vi "Win_Handler.vi"() -> ()   [LabVIEW 2025]
panel:
  out "Error Out":errorcluster
  in  "Error In":errorcluster
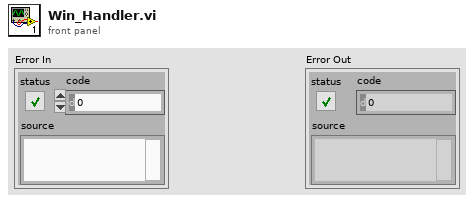
[diagram p1: front panel]
types:
  T1 = typedef "Queue_Data.ctl" = cluster{"CMD":string, "Data":variant}
  T2 = typedef "IMAQ Image.ctl" = refnum<image>
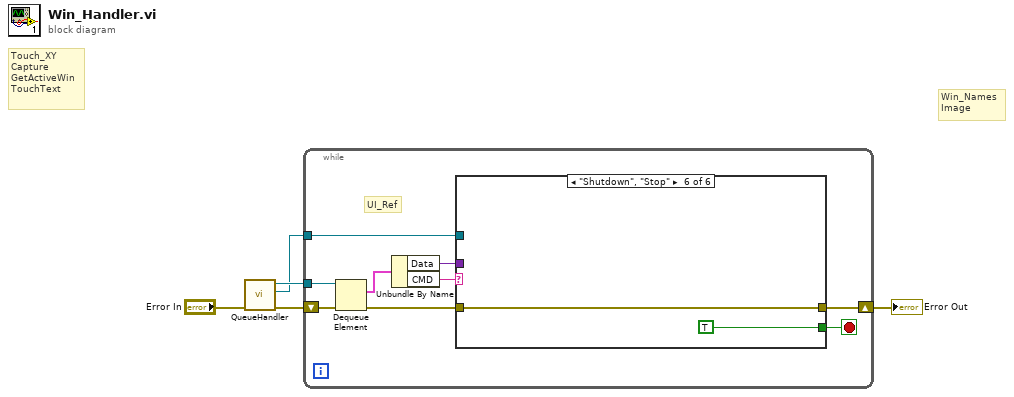
[diagram p0: block diagram]
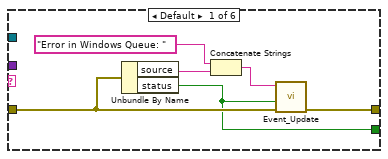
[diagram p2: hidden frame]
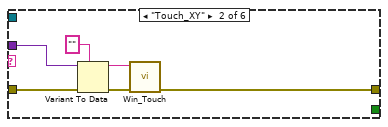
[diagram p3: hidden frame]
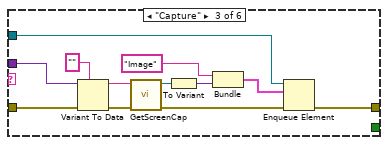
[diagram p4: hidden frame]
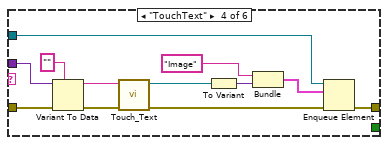
[diagram p5: hidden frame]
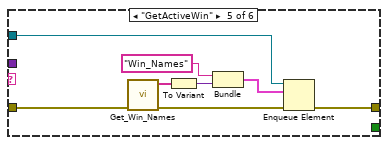
[diagram p6: hidden frame]
diagram:
  # "Win_Names\nImage"
  # "Touch_XY\nCapture\nGetActiveWin\nTouchText"
  n1 = call "QueueHandler.vi"("Error In"="Error In") -> ("Error Out"=w4:errorcluster, "UI"=w1:refnum<queue>, "Win"=w2:refnum<queue>)  [unwired: 8 in]
  n2 = while {
    tunnel: w2 -> [w14]
    shift-right: [w7] -> w5
    shift-left: w4 -> [w13]
    tunnel: w1 -> [w6]
    stop <- w9 stop-if-true
    # "UI_Ref"
    n3 = Dequeue Element(queue=w14, error in (no error)=w13) -> (element=w11:T1, error out=w12:errorcluster)  [unwired: 1 in, 2 out]
    n4 = Unbundle By Name(w11) -> ("Data"=w8:variant, "CMD"=w10:string)
    n5 = case shown="\"Shutdown\", \"Stop\"" w10 {
      tunnel: w12 -> [w19 w24 w37 w49 w58 w60]
      tunnel: [w20 w26 w31 w46 w56 w60] -> w7
      tunnel: [w15 _ _ _ _ TRUE ("status")] -> w9
      tunnel: w8 -> [_ w25 w38 w50 _ _]
      tunnel: w6 -> [_ _ w33 w47 w57 _]
      frame Default {
        n6 = Unbundle By Name(w19) -> ("source"=w17:string, "status"=w15:bool)
        n7 = Concatenate Strings("Error in Windows Queue: ", w17) -> (w18:string)
        n8 = call "Event_Update.vi"("Error In"=w19, "Update?"=w15, "Event"=w18) -> ("Error Out"=w20:errorcluster)  [unwired: 8 in]
      }
      frame "Touch_XY" {
        n9 = Variant To Data(error in=w24, type="", Variant=w25) -> (data=w21:string, error out=w23:errorcluster)
        n10 = call "Win_Touch.vi"("error in (no error)"=w23, "TouchXY"=w21) -> ("error out"=w26:errorcluster)  [unwired: 9 in]
      }
      frame "Capture" {
        n11 = Variant To Data(error in=w37, type="", Variant=w38) -> (data=w34:string, error out=w35:errorcluster)
        n12 = call "GetScreenCap.vi"("error in (no error)"=w35, "Win Name"=w34) -> ("error out"=w32:errorcluster, "Image Out"=w29:T2)  [unwired: 8 in]
        n13 = To Variant(anything=w29) -> (Variant=w28:variant)
        n14 = Bundle("Image", "Variant"=w28) -> (w27:cluster{string, "Variant":variant})  [unwired: 1 in]
        n15 = Enqueue Element(queue=w33, element=w27, error in (no error)=w32) -> (error out=w31:errorcluster)  [unwired: 1 in, 2 out]
      }
      frame "TouchText" {
        n16 = Variant To Data(error in=w49, type="", Variant=w50) -> (data=w41:string, error out=w42:errorcluster)
        n17 = call "Touch_Text.vi"("Error In"=w42, "TextTouch"=w41) -> ("error out"=w39:errorcluster, "Image"=w40:T2)  [unwired: 8 in]
        n18 = To Variant(anything=w40) -> (Variant=w44:variant)
        n19 = Bundle("Image", "Variant"=w44) -> (w43:cluster{string, "Variant":variant})  [unwired: 1 in]
        n20 = Enqueue Element(queue=w47, element=w43, error in (no error)=w39) -> (error out=w46:errorcluster)  [unwired: 1 in, 2 out]
      }
      frame "GetActiveWin" {
        n21 = call "Get_Win_Names.vi"("error in"=w58) -> ("Win_Names"=w51:string[], "error out"=w52:errorcluster)  [unwired: 8 in]
        n22 = To Variant(anything=w51) -> (Variant=w54:variant)
        n23 = Bundle("Win_Names", "Variant"=w54) -> (w53:cluster{string, "Variant":variant})  [unwired: 1 in]
        n24 = Enqueue Element(queue=w57, element=w53, error in (no error)=w52) -> (error out=w56:errorcluster)  [unwired: 1 in, 2 out]
      }
      frame "Shutdown", "Stop" {
      }
    }
  }
  "Error Out" <- w5
